vi "to string.vi"(8 "error in":errorcluster, 11 "Scan Engine configuration in":refnum<class "Scan Engine configuration.lvclass">) -> (0 "error out":errorcluster, 1 "data":string, 2 "version":string, 3 "Scan Engine configuration out":refnum<class "Scan Engine configuration.lvclass">)   [LabVIEW 2014, in "Scan Engine configuration.lvclass"]
doc: "Provides an interface for saving a module configuration to a file or other serialized data source. It is recommended that all children of this class store data in two sets--data required for its own initialization, and any data required for parent initialization--and that each implementation uses the <b>Call Parent Method</b> primitive to serialize parent information."
uses:
  Scan Engine configuration.lvclass
  Scan Engine configuration.lvclass/Scan Engine configuration.ctl
  current version.vi
  <vilib>/NI/Tag Bus Module Framework/module configuration/TBM module configuration.lvclass
  <vilib>/NI/Configuration Framework/serializable configuration/NISE_CEF_serializable configuration.lvclass
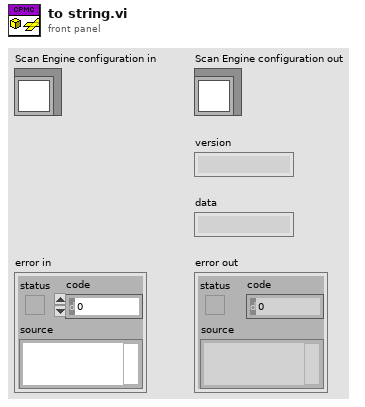
[diagram p1: front panel]
types:
  T1 = typedef "Scan Engine configuration.lvclass/Line.ctl" = cluster{"channel":refnum<class "TBM channel.lvclass">, "Tag":string}
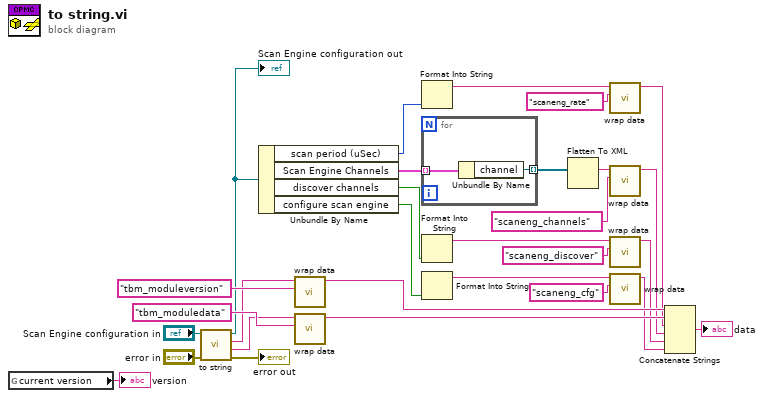
[diagram p0: block diagram]
diagram:
  n1 = global read "current version.vi" "current version"() -> (→"version":string)
  n2 = call-parent "to string.vi"("error in"="error in", "module configuration in"="Scan Engine configuration in") -> ("error out"=→"error out":errorcluster, "data"=w22:string, "version"=w23:string, "module configuration out"=w17:refnum<class "Scan Engine configuration.lvclass">)  [unwired: 6 in]
  "Scan Engine configuration out" <- w17
  n3 = Unbundle By Name(w17) -> ("scan period (uSec)"=w16:u32, "Scan Engine Channels"=w2:T1[], "discover channels"=w11:bool, "configure scan engine"=w10:bool)
  n4 = call <vilib>:"wrap data.vi"("identifier"="tbm_moduleversion" ("additional identifier"), "data to wrap"=w23) -> ("wrapped data"=w24:string)  [unwired: 9 in]
  n5 = call <vilib>:"wrap data.vi"("identifier"="tbm_moduledata" ("additional identifier"), "data to wrap"=w22) -> ("wrapped data"=w7:string)  [unwired: 9 in]
  n6 = Format Into String(w16) -> (resulting string=w15:string)  [unwired: 3 in, 1 out]
  n7 = for {
    tunnel: w2 -> [w31] mode=indexing
    tunnel: [w30] -> w1 mode=indexing
    n8 = Unbundle By Name(w31) -> ("channel"=w30:refnum<class "TBM channel.lvclass">)
  }
  n9 = Format Into String(w11) -> (resulting string=w9:string)  [unwired: 3 in, 1 out]
  n10 = Format Into String(w10) -> (resulting string=w8:string)  [unwired: 3 in, 1 out]
  n11 = Flatten To XML(anything=w1) -> (xml string=w18:string)
  n12 = call <vilib>:"wrap data.vi"("identifier"="scaneng_rate", "data to wrap"=w15) -> ("wrapped data"=w6:string)  [unwired: 9 in]
  n13 = call <vilib>:"wrap data.vi"("identifier"="scaneng_channels" ("additional identifier"), "data to wrap"=w18) -> ("wrapped data"=w5:string)  [unwired: 9 in]
  n14 = call <vilib>:"wrap data.vi"("identifier"="scaneng_discover", "data to wrap"=w9) -> ("wrapped data"=w4:string)  [unwired: 9 in]
  n15 = call <vilib>:"wrap data.vi"("identifier"="scaneng_cfg", "data to wrap"=w8) -> ("wrapped data"=w3:string)  [unwired: 9 in]
  n16 = Concatenate Strings(w24, w7, w6, w5, w4, w3) -> (→"data":string)
